vi "Facade.vi"(0 "Data In":T8 {"Duration (s)" format="%<%M:%S>T"}, 2 "Display State In":T6, 3 "Container State":T7) -> (6 "Data Out":T8 {"Duration (s)" format="%<%M:%S>T"}, 7 "Display State Out":T6, 8 "Action":T5)   [LabVIEW 2015, in "Song Queue.lvlib" / "Song Queue.xctl"]
uses:
  Song Queue.xctl
  Data.ctl
  controls/Queue Song Display.ctl
  file/MusicElement/Song/Song Duration.ctl
  controls/Dequeue Control.ctl
  <vilib>/_xctls/Container State.ctl
  State.ctl
  <vilib>/_xctls/Action.ctl
  controls/Ascending_Descending Order.ctl
  controls/Enqueue Control.ctl
  file/MusicElement/MusicElementLibrary/SongLibrary/Song Display Sort Option.ctl
  <vilib>/_xctls/XControlSupport.lvlib
  file/MusicElement/MusicElementLibrary/SongLibrary/SongLibrary.lvclass
  file/MusicElement/Song/Song.lvclass
panel:
  in  "Remove Filters":bool
  in  "Time Sort":bool
  out "Sort Time Indicator":T1
  out "Sort Album Indicator":T1
  in  "Album Sort":bool
  out "Sort Artist Indicator":T1
  in  "Artist Sort":bool
  in  "Song Sort":bool
  out "Sort Songs Indicator":T1
  out "Unfiltered Array":T2[](array[typedef]) {"Duration (s)" format="%<%M:%S>T"}
  in  "Array":T2[](array[typedef]) {"Duration (s)" format="%<%M:%S>T"}
  in  "Scrollbar":i32(c297)
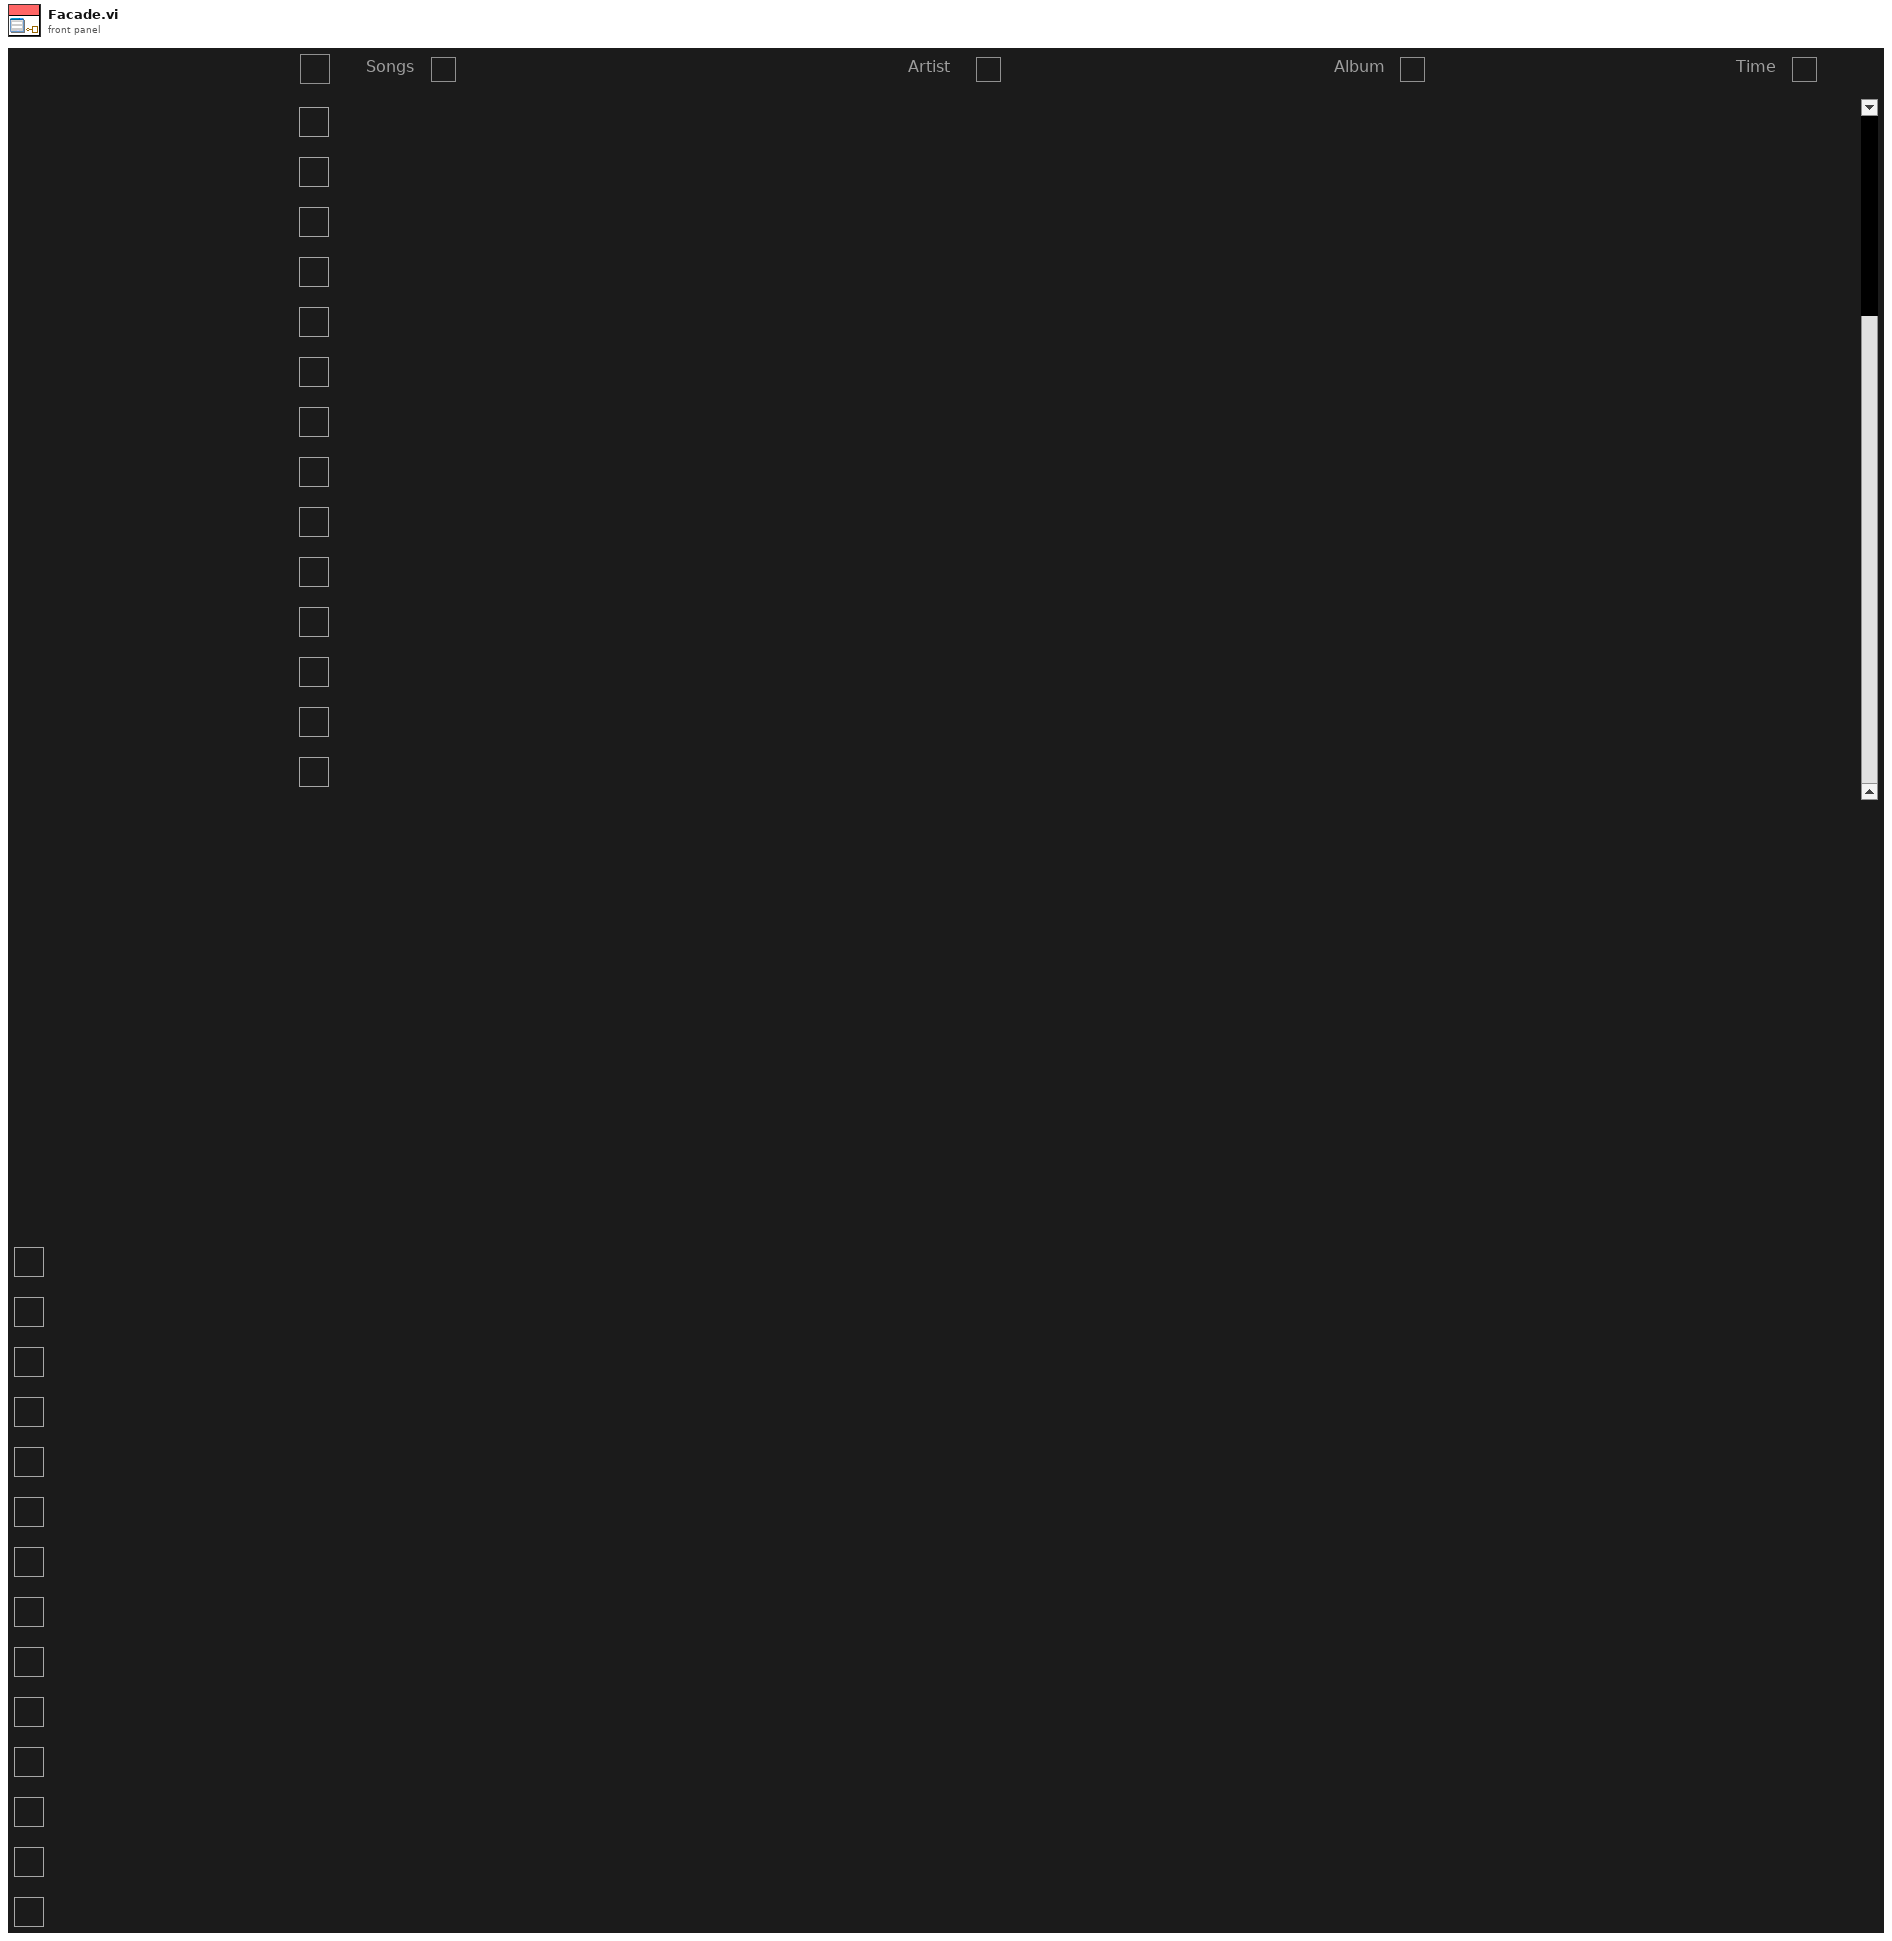
[diagram p1: front panel]
types:
  T1 = typedef "Ascending_Descending Order.ctl" = bool
  T2 = typedef "Queue Song Display.ctl" = cluster{"Song Name":string, "Artist":string, "Album":string, "Duration (s)":T3, "UID":string, "Dequeue":T4}
  T3 = typedef "Song.lvclass/Song Duration.ctl" = timestamp
  T4 = typedef "Dequeue Control.ctl" = bool
  T5 = typedef "XControlSupport.lvlib/Action.ctl" = cluster{"Data Changed?":bool, "State Changed?":bool, "Action Name":string}
  T6 = typedef "Song Queue.lvlib/Song Queue.xctl/State.ctl" = cluster{"Element Selected Event":refnum<user-event>}
  T7 = typedef "XControlSupport.lvlib/Container State.ctl" = cluster{"Indicator?":bool, "Run Mode?":bool, " Refnum":refnum<vi>}
  T8 = typedef "Song Queue.lvlib/Song Queue.xctl/Data.ctl" = T2[]
  T9 = typedef "Enqueue Control.ctl" = bool
  T10 = cluster{"Song Name":bool, "Artist":bool, "Album":bool, "Duration (s)":bool, "UID":bool, "Enqueue":T9}
  T11 = typedef "SongLibrary.lvclass/Song Display Sort Option.ctl" = enum16{"Song", "Artist", "Album", "Time"}
  T12 = cluster{"Song Name":bool, "Artist":bool, "Album":bool, "Duration (s)":bool, "UID":bool, "Dequeue":T4}[]
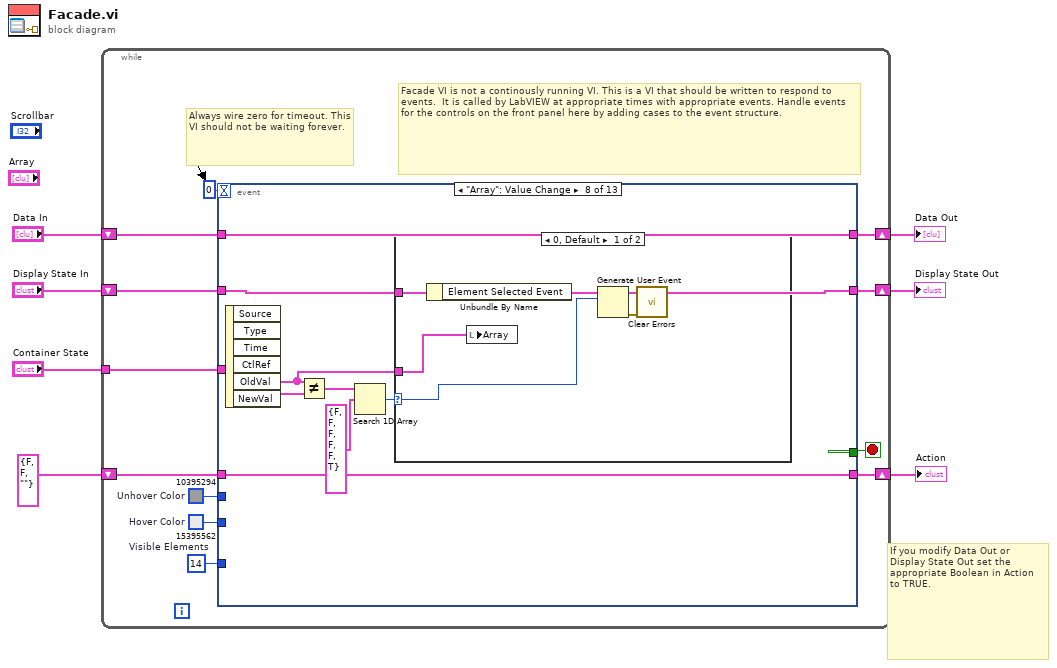
[diagram p0: block diagram]
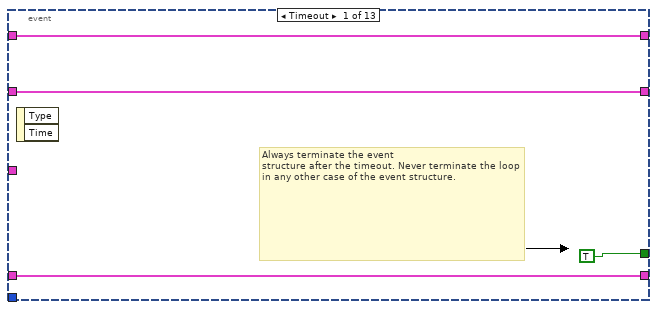
[diagram p2: hidden frame]
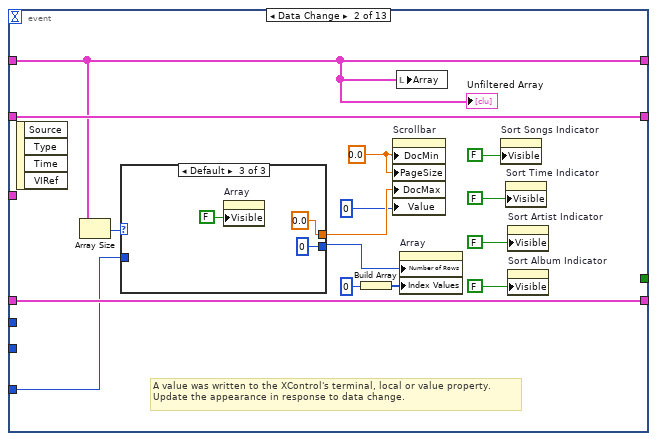
[diagram p3: hidden frame]
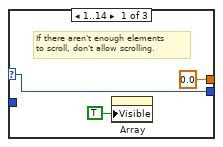
[diagram p4: hidden frame]
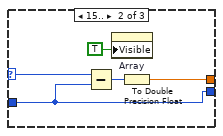
[diagram p5: hidden frame]
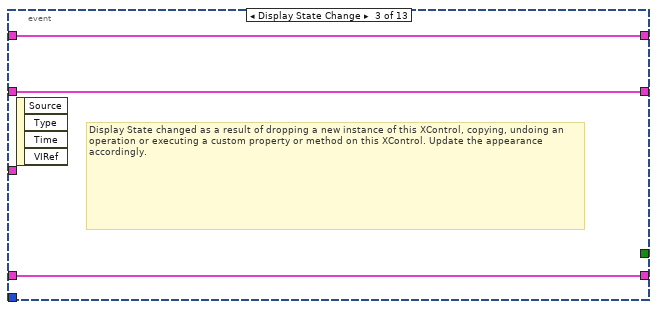
[diagram p6: hidden frame]
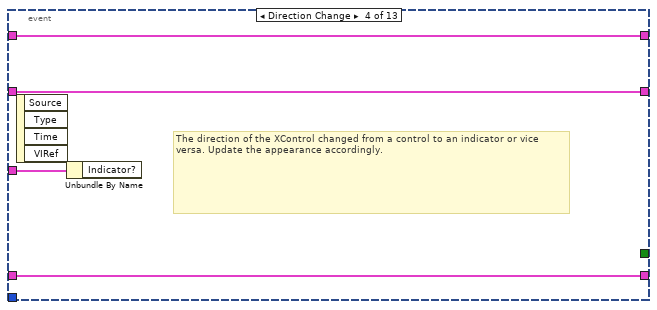
[diagram p7: hidden frame]
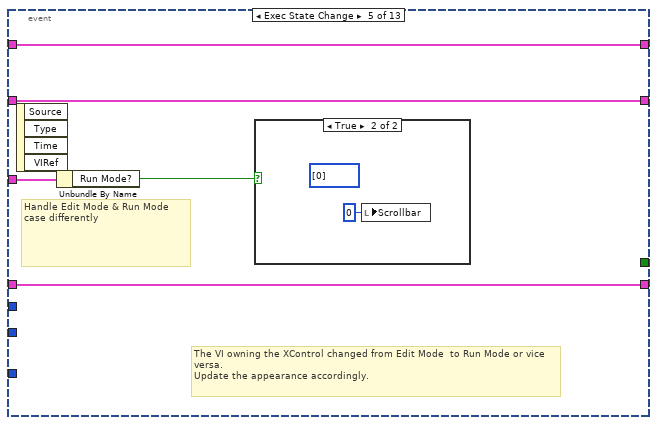
[diagram p8: hidden frame]
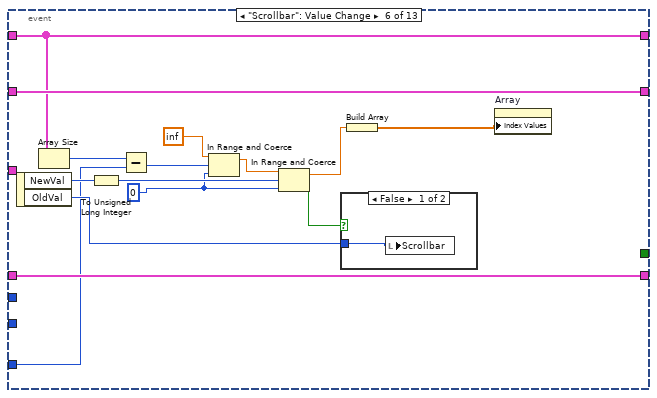
[diagram p10: hidden frame]
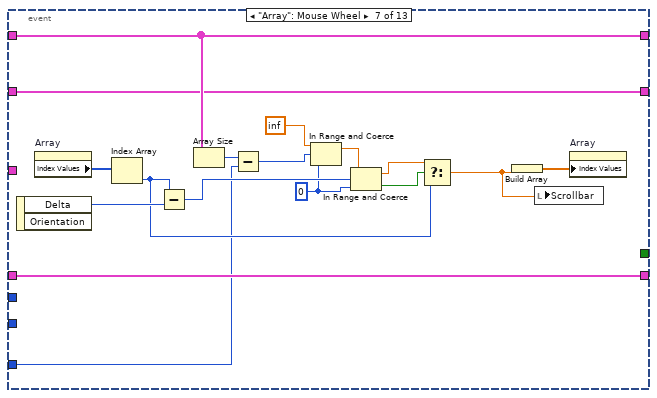
[diagram p12: hidden frame]
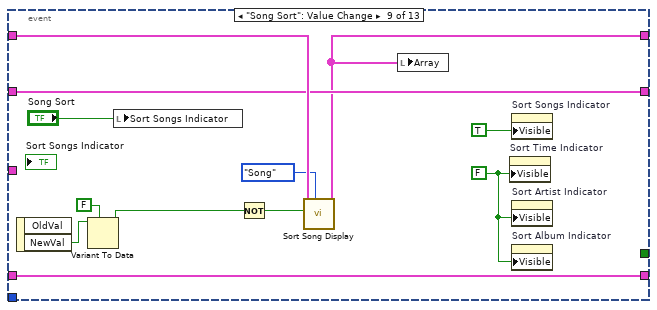
[diagram p14: hidden frame]
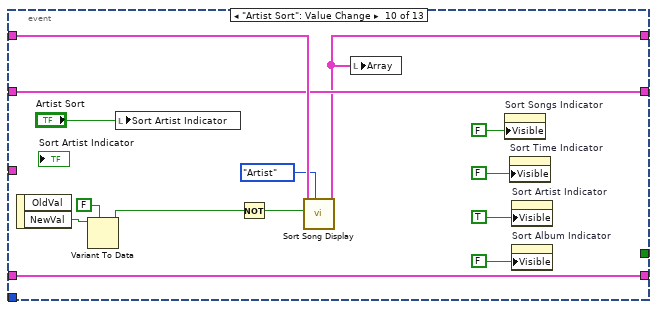
[diagram p15: hidden frame]
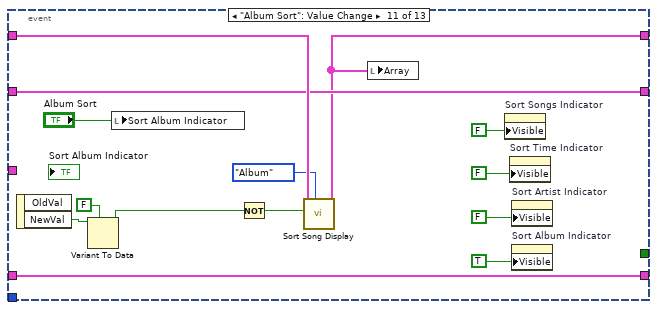
[diagram p16: hidden frame]
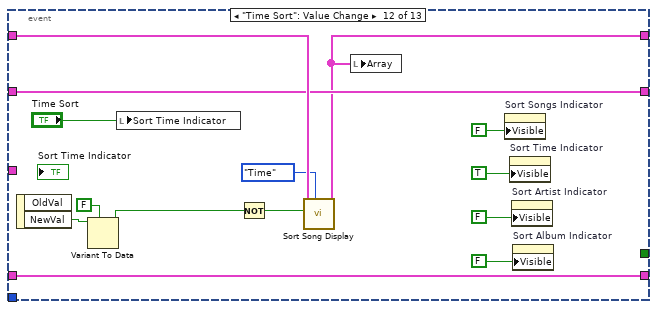
[diagram p17: hidden frame]
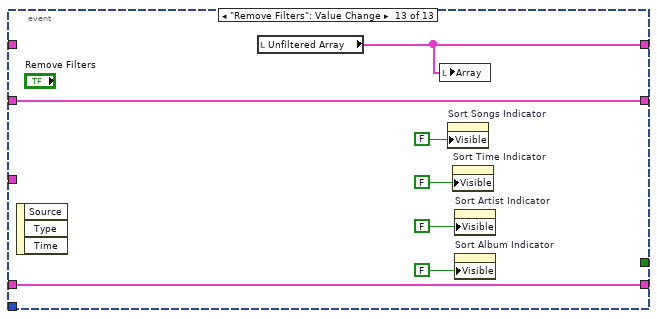
[diagram p18: hidden frame]
diagram:
  # "If you modify Data Out or\nDisplay State Out set the\nappropriate Boolean in Action\nto TRUE."
  n1 = while {
    shift-right: [w18] -> w3
    shift-left: "Display State In" -> [w19]
    tunnel: "Container State" -> [w15]
    shift-right: [w13] -> w2
    shift-left: "Data In" -> [w14]
    shift-right: [w11] -> w1
    shift-left: T5 {"Data Changed?"=FALSE, "State Changed?"=FALSE, "Action Name"=""} ("Action") -> [w12]
    stop <- w17 stop-if-true
    w8 = u32 15395562  # Hover Color
    w9 = u32 10395294  # Unhover Color
    w10 = 14  # Visible Elements
    # "Facade VI is not a continously running VI. This is a VI that should be written to respond to events.  It is called by LabVIEW at appropriate times with appropriate events. Handle events for the controls on the front panel here by adding cases to the event structure."
    # "Always wire zero for timeout. This\nVI should not be waiting forever."
    n2 = event shown="[7] \"Array\": Value Change" {
      selector: _ -> [_ _ _ _ _ _ _ _ _ _ _ _ _]
      dyn-events: _ -> [_ _ _ _ _ _ _ _ _ _ _ _ _]
      timeout: 0 -> [_ _ _ _ _ _ _ _ _ _ _ _ _]
      tunnel: w19 -> [w21 w28 w52 w55 w60 w75 w90 w98 w116 w131 w145 w159 w169]
      tunnel: [w21 w28 w52 w55 w60 w75 w90 w98 w116 w131 w145 w159 w169] -> w18
      tunnel: [TRUE _ _ _ _ _ _ _ _ _ _ _ _] -> w17
      tunnel: w15 -> [_ _ _ w56 w61 _ _ _ _ _ _ _ _]
      tunnel: w14 -> [w20 w27 w51 w54 w59 w73 w91 w103 w120 w134 w148 w162 _]
      tunnel: [w20 w27 w51 w54 w59 w73 w91 w103 w110 w121 w135 w149 w163] -> w13
      tunnel: [w22 w38 w50 w53 w58 w76 w92 w102 w115 w130 w144 w158 w168] -> w11
      tunnel: w12 -> [w22 w38 w50 w53 w58 w76 w92 w102 w115 w130 w144 w158 w168]
      tunnel: w10 -> [_ w36 _ _ _ w68 w86 _ _ _ _ _ _]
      tunnel: w9 -> [_ _ _ _ _ _ _ _ _ _ _ _ _]
      tunnel: w8 -> [_ _ _ _ _ _ _ _ _ _ _ _ _]
      event Timeout {
        # "Always terminate the event\nstructure after the timeout. Never terminate the loop in any other case of the event structure."
        n3 = event-data() -> ()  [unwired: 1 in, 2 out]
      }
      event Data Change {
        w31 = 0.0 ("Doc Min")
        # "A value was written to the XControl's terminal, local or value property.\nUpdate the appearance in response to data change."
        n4 = event-data() -> ()  [unwired: 1 in, 4 out]
        n5 = Array Size(array=w27) -> (size(s)=w37:i32)
        n6 = case shown="Default" w37 {
          selector: w37 -> [w41 w45 _]
          tunnel: [w41 w43 0 ("y")] -> w29
          tunnel: [0.0 ("Doc Min") w46 0.0 ("Doc Max")] -> w30
          tunnel: w36 -> [_ w43 _]
          frame 1..14 {
            # "If there aren't enough elements\nto scroll, don't allow scrolling."
            n7 = property on="Array" class="Arr"("Visible"=TRUE) -> ()  [unwired: 2 in, 2 out]
          }
          frame 15.. {
            n8 = Subtract(x=w45, y=w43) -> (x-y=w44:i32)
            n9 = property on="Array" class="Arr"("Visible"=TRUE) -> ()  [unwired: 2 in, 2 out]
            n10 = To Double Precision Float(number=w44) -> (double precision float=w46:dbl)
          }
          frame Default {
            n11 = property on="Array" class="Arr"("Visible"=FALSE) -> ()  [unwired: 2 in, 2 out]
          }
        }
        n12 = Build Array(0 ("y")) -> (w25:i32[])
        n13 = property on="Scrollbar" class="Scroll (strict)"("DocMin"=w31, "PageSize"=w31, "DocMax"=w30, "Value"=0 ("y")) -> ()  [unwired: 2 in, 2 out]
        n14 = local write "Array"(w27) -> ()
        n15 = property on="Array" class="Arr"("Number of Rows"=w29, "Index Values"=w25) -> ()  [unwired: 2 in, 2 out]
        n16 = property on="Sort Songs Indicator" class="Bool (strict)"("Visible"=FALSE) -> ()  [unwired: 2 in, 2 out]
        n17 = property on="Sort Time Indicator" class="Bool (strict)"("Visible"=FALSE) -> ()  [unwired: 2 in, 2 out]
        n18 = property on="Sort Artist Indicator" class="Bool (strict)"("Visible"=FALSE) -> ()  [unwired: 2 in, 2 out]
        n19 = property on="Sort Album Indicator" class="Bool (strict)"("Visible"=FALSE) -> ()  [unwired: 2 in, 2 out]
        "Unfiltered Array" <- w27
      }
      event Display State Change {
        # "Display State changed as a result of dropping a new instance of this XControl, copying, undoing an operation or executing a custom property or method on this XControl. Update the appearance accordingly."
        n20 = event-data() -> ()  [unwired: 1 in, 4 out]
      }
      event Direction Change {
        # "The direction of the XControl changed from a control to an indicator or vice versa. Update the appearance accordingly."
        n21 = event-data() -> ()  [unwired: 1 in, 4 out]
        n22 = Unbundle By Name(w56) -> ()  [unwired: 1 out]
      }
      event Exec State Change {
        # "The VI owning the XControl changed from Edit Mode  to Run Mode or vice versa.\nUpdate the appearance accordingly."
        # "Handle Edit Mode & Run Mode\ncase differently"
        n23 = event-data() -> ()  [unwired: 1 in, 4 out]
        n24 = Unbundle By Name(w61) -> ("Run Mode?"=w57:bool)
        n25 = case shown="True" w57 {
          frame False {
          }
          frame True {
            (unwired) u32[] [0] ("Index Values")
            n26 = local write "Scrollbar"(0 ("Scrollbar")) -> ()
          }
        }
      }
      event "Scrollbar": Value Change {
        w64 = u32 0 ("upper limit")
        n27 = event-data() -> ("NewVal"=w77:i32, "OldVal"=w69:i32)  [unwired: 1 in]
        n28 = Array Size(array=w73) -> (size(s)=w72:i32)
        n29 = To Unsigned Long Integer(number=w77) -> (unsigned 32bit integer=w74:u32)
        n30 = Subtract(x=w72, y=w68) -> (x-y=w66:i32)
        n31 = In Range and Coerce(upper limit=inf, x=w66, lower limit=w64) -> (coerced(x)=w63:dbl)  [unwired: 1 out]
        n32 = In Range and Coerce(upper limit=w63, x=w74, lower limit=w64) -> (coerced(x)=w71:dbl, In Range?=w70:bool)
        n33 = case shown="False" w70 {
          tunnel: w69 -> [w78 _]
          frame False {
            n34 = local write "Scrollbar"(w78) -> ()
          }
          frame True {
          }
        }
        n35 = Build Array(w71) -> (w67:dbl[])
        n36 = property on="Array" class="Arr"("Index Values"=w67) -> ()  [unwired: 2 in, 2 out]
      }
      event "Array": Mouse Wheel {
        w81 = u32 0 ("upper limit")
        n37 = event-data() -> ("Delta"=w95:i32)  [unwired: 1 in, 1 out]
        n38 = property on="Array" class="Arr"() -> ("Index Values"=w83:u32[])  [unwired: 2 in, 2 out]
        n39 = Index Array(array=w83) -> (element=w87:u32)  [unwired: 1 in]
        n40 = Subtract(x=w87, y=w95) -> (x-y=w93:u32)
        n41 = Array Size(array=w91) -> (size(s)=w94:i32)
        n42 = Subtract(x=w94, y=w86) -> (x-y=w80:i32)
        n43 = In Range and Coerce(upper limit=inf, x=w80, lower limit=w81) -> (coerced(x)=w79:dbl)  [unwired: 1 out]
        n44 = In Range and Coerce(upper limit=w79, x=w93, lower limit=w81) -> (coerced(x)=w88:dbl, In Range?=w89:bool)
        n45 = Select(t=w88, s=w89, f=w87) -> (s? t:f=w85:dbl)
        n46 = Build Array(w85) -> (w84:dbl[])
        n47 = local write "Scrollbar"(w85) -> ()
        n48 = property on="Array" class="Arr"("Index Values"=w84) -> ()  [unwired: 2 in, 2 out]
      }
      event "Array": Value Change {
        n49 = event-data() -> ("OldVal"=w96:T2[], "NewVal"=w97:T2[])  [unwired: 1 in, 4 out]
        n50 = Not Equal?(x=w96, y=w97) -> (x != y?=w101:T12)
        n51 = Search 1D Array(1D array=w101, element=T10 {"Song Name"=FALSE, "Artist"=FALSE, "Album"=FALSE, "Duration (s)"=FALSE, "UID"=FALSE, "Enqueue"=TRUE}) -> (index of element=w100:i32)  [unwired: 1 in]
        n52 = case shown="0, Default" w100 {
          selector: w100 -> [w104 _]
          tunnel: w98 -> [w108 _]
          tunnel: w96 -> [w105 _]
          frame 0, Default {
            n53 = Unbundle By Name(w108) -> ("Element Selected Event"=w106:refnum<user-event>)
            n54 = local write "Array"(w105) -> ()
            n55 = Generate User Event(user event=w106, event data cluster=w104) -> (error out=w107:errorcluster)  [unwired: 2 in, 1 out]
            n56 = call <vilib>:"Clear Errors.vi"("error in (no error)"=w107) -> ()  [unwired: 5 in, 2 out]
          }
          frame ..-1 {
          }
        }
      }
      event "Song Sort": Value Change {
        w113 = FALSE ("Visible")
        n57 = event-data() -> ("NewVal"=w111:bool)  [unwired: 1 in, 1 out]
        n58 = Variant To Data(type=T1 FALSE ("Sort Songs Indicator"), Variant=w111) -> (data=w109:T1)  [unwired: 1 in, 1 out]
        n59 = local write "Sort Songs Indicator"("Song Sort") -> ()
        n60 = Not(x=w109) -> (.not. x?=w112:T1)
        n61 = call "Sort Song Display.vi"("Options"=Song_Display_Sort_Option."Song", "Reverse?"=w112, "Songs"=w120) -> ("Sorted Songs"=w110:T2[])  [unwired: 7 in, 1 out]
        n62 = local write "Array"(w110) -> ()
        n63 = property on="Sort Time Indicator" class="Bool (strict)"("Visible"=w113) -> ()  [unwired: 2 in, 2 out]
        n64 = property on="Sort Songs Indicator" class="Bool (strict)"("Visible"=TRUE) -> ()  [unwired: 2 in, 2 out]
        n65 = property on="Sort Artist Indicator" class="Bool (strict)"("Visible"=w113) -> ()  [unwired: 2 in, 2 out]
        n66 = property on="Sort Album Indicator" class="Bool (strict)"("Visible"=w113) -> ()  [unwired: 2 in, 2 out]
      }
      event "Artist Sort": Value Change {
        n67 = event-data() -> ("NewVal"=w122:bool)  [unwired: 1 in, 1 out]
        n68 = Variant To Data(type=T1 FALSE ("Sort Songs Indicator"), Variant=w122) -> (data=w127:T1)  [unwired: 1 in, 1 out]
        n69 = local write "Sort Artist Indicator"("Artist Sort") -> ()
        n70 = Not(x=w127) -> (.not. x?=w128:T1)
        n71 = call "Sort Song Display.vi"("Options"=Song_Display_Sort_Option."Artist", "Reverse?"=w128, "Songs"=w134) -> ("Sorted Songs"=w121:T2[])  [unwired: 7 in, 1 out]
        n72 = local write "Array"(w121) -> ()
        n73 = property on="Sort Songs Indicator" class="Bool (strict)"("Visible"=FALSE) -> ()  [unwired: 2 in, 2 out]
        n74 = property on="Sort Time Indicator" class="Bool (strict)"("Visible"=FALSE) -> ()  [unwired: 2 in, 2 out]
        n75 = property on="Sort Artist Indicator" class="Bool (strict)"("Visible"=TRUE) -> ()  [unwired: 2 in, 2 out]
        n76 = property on="Sort Album Indicator" class="Bool (strict)"("Visible"=FALSE) -> ()  [unwired: 2 in, 2 out]
      }
      event "Album Sort": Value Change {
        n77 = event-data() -> ("NewVal"=w138:bool)  [unwired: 1 in, 1 out]
        n78 = Variant To Data(type=T1 FALSE ("Sort Songs Indicator"), Variant=w138) -> (data=w141:T1)  [unwired: 1 in, 1 out]
        n79 = local write "Sort Album Indicator"("Album Sort") -> ()
        n80 = Not(x=w141) -> (.not. x?=w142:T1)
        n81 = call "Sort Song Display.vi"("Options"=Song_Display_Sort_Option."Album", "Reverse?"=w142, "Songs"=w148) -> ("Sorted Songs"=w135:T2[])  [unwired: 7 in, 1 out]
        n82 = local write "Array"(w135) -> ()
        n83 = property on="Sort Songs Indicator" class="Bool (strict)"("Visible"=FALSE) -> ()  [unwired: 2 in, 2 out]
        n84 = property on="Sort Time Indicator" class="Bool (strict)"("Visible"=FALSE) -> ()  [unwired: 2 in, 2 out]
        n85 = property on="Sort Artist Indicator" class="Bool (strict)"("Visible"=FALSE) -> ()  [unwired: 2 in, 2 out]
        n86 = property on="Sort Album Indicator" class="Bool (strict)"("Visible"=TRUE) -> ()  [unwired: 2 in, 2 out]
      }
      event "Time Sort": Value Change {
        n87 = event-data() -> ("NewVal"=w153:bool)  [unwired: 1 in, 1 out]
        n88 = Variant To Data(type=T1 FALSE ("Sort Songs Indicator"), Variant=w153) -> (data=w155:T1)  [unwired: 1 in, 1 out]
        n89 = local write "Sort Time Indicator"("Time Sort") -> ()
        n90 = Not(x=w155) -> (.not. x?=w156:T1)
        n91 = call "Sort Song Display.vi"("Options"=Song_Display_Sort_Option."Time", "Reverse?"=w156, "Songs"=w162) -> ("Sorted Songs"=w149:T2[])  [unwired: 7 in, 1 out]
        n92 = local write "Array"(w149) -> ()
        n93 = property on="Sort Songs Indicator" class="Bool (strict)"("Visible"=FALSE) -> ()  [unwired: 2 in, 2 out]
        n94 = property on="Sort Time Indicator" class="Bool (strict)"("Visible"=TRUE) -> ()  [unwired: 2 in, 2 out]
        n95 = property on="Sort Artist Indicator" class="Bool (strict)"("Visible"=FALSE) -> ()  [unwired: 2 in, 2 out]
        n96 = property on="Sort Album Indicator" class="Bool (strict)"("Visible"=FALSE) -> ()  [unwired: 2 in, 2 out]
      }
      event "Remove Filters": Value Change {
        n97 = event-data() -> ()  [unwired: 1 in, 3 out]
        n98 = local read "Unfiltered Array"() -> (w163:T2[])
        n99 = local write "Array"(w163) -> ()
        n100 = property on="Sort Songs Indicator" class="Bool (strict)"("Visible"=FALSE) -> ()  [unwired: 2 in, 2 out]
        n101 = property on="Sort Time Indicator" class="Bool (strict)"("Visible"=FALSE) -> ()  [unwired: 2 in, 2 out]
        n102 = property on="Sort Artist Indicator" class="Bool (strict)"("Visible"=FALSE) -> ()  [unwired: 2 in, 2 out]
        n103 = property on="Sort Album Indicator" class="Bool (strict)"("Visible"=FALSE) -> ()  [unwired: 2 in, 2 out]
      }
    }
  }
  "Display State Out" <- w3
  "Data Out" <- w2
  "Action" <- w1
